vi "test.vi"() -> ()   [LabVIEW 2023]
uses:
  <vilib>/numeric/Random Number (Range) U64.vi
panel:
  out "Numeric":dbl
  in  "Boolean":bool
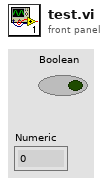
[diagram p1: front panel]
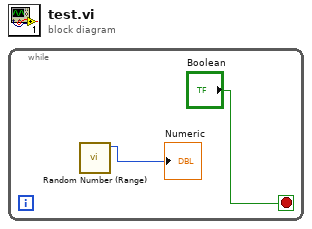
[diagram p0: block diagram]
diagram:
  n1 = while {
    stop <- "Boolean" stop-if-true
    n2 = call-poly <vilib>:"Random Number (Range).vi"() -> ("number"=→"Numeric":u64)  [unwired: 11 in]
  }
